vi "img_open_file.vi"(8 "error in":errorcluster, 10 "Operation (open)":enum16{"Open", "Create/Replace"}(ring), 11 "Filename":path) -> (0 "error out":errorcluster, 1 "lpBytesPerSector":u32, 2 "lpFileSize":u64, 3 "hFile":i64)   [LabVIEW 2016]
doc: "This Vi opens a file handle for unbuffered reading or writing.\n\nhFile: File handle\n\nlpFileSize: Returns the file size in bytes. Use for reading back data.\n\nlpBytesPerSector: Returns the number of bytes per sector for the hard drive array. Unbuffered reads and writes must be a multiple of the disk sector size."
uses:
  kernel32.dll
panel:
  in  "Access (read/write)":enum16{"read/write", "read-only", "write-only"}(ring)
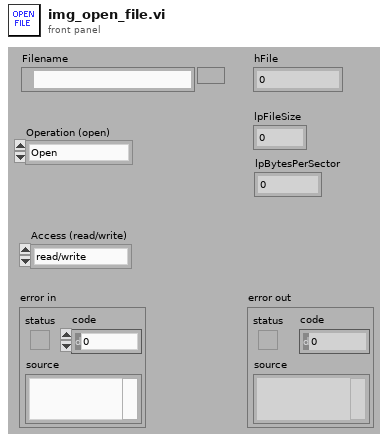
[diagram p1: front panel]
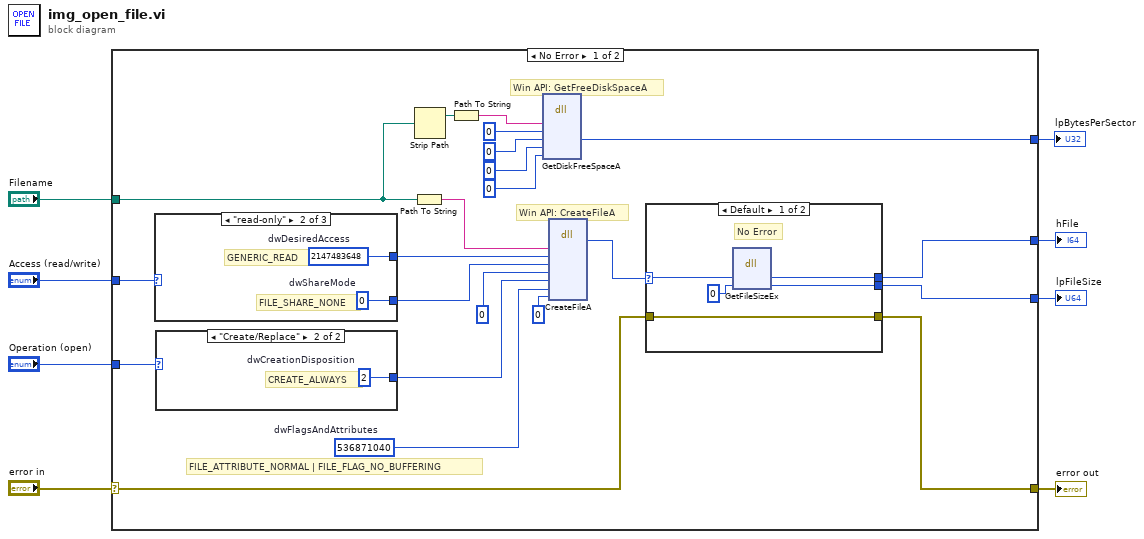
[diagram p0: block diagram]
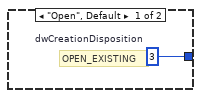
[diagram p2: hidden frame]
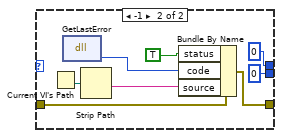
[diagram p3: hidden frame]
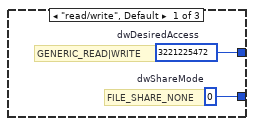
[diagram p4: hidden frame]
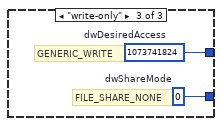
[diagram p5: hidden frame]
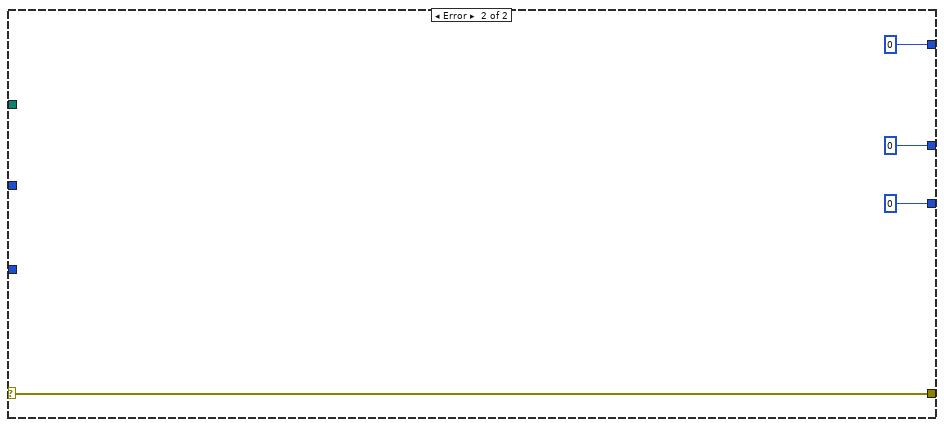
[diagram p6: hidden frame]
diagram:
  n1 = case shown="No Error" "error in" {
    selector: "error in" -> [w25 w53]
    tunnel: [w15 u32 0 ("hFile")] -> w8
    tunnel: "Filename" -> [w18 _]
    tunnel: [w26 w53] -> w6
    tunnel: "Operation (open)" -> [w11 _]
    tunnel: [w14 u64 0 ("lpFileSize")] -> w4
    tunnel: [w19 u32 0 ("lpBytesPerSector")] -> w2
    tunnel: "Access (read/write)" -> [w12 _]
    frame No Error {
      w30 = u32 536871040  # dwFlagsAndAttributes
      # "Win API: GetFreeDiskSpaceA"
      # "FILE_ATTRIBUTE_NORMAL | FILE_FLAG_NO_BUFFERING"
      # "Win API: CreateFileA"
      n2 = case shown="\"read-only\"" w12 {
        tunnel: [w46 w48 w51] -> w28
        tunnel: [w47 w49 w50] -> w27
        frame "read/write", Default {
          w46 = u32 0  # dwShareMode
          w47 = u32 3221225472  # dwDesiredAccess
          # "FILE_SHARE_NONE"
          # "GENERIC_READ|WRITE"
        }
        frame "read-only" {
          w48 = u32 0  # dwShareMode
          w49 = u32 2147483648  # dwDesiredAccess
          # "FILE_SHARE_NONE"
          # "GENERIC_READ"
        }
        frame "write-only" {
          w51 = u32 0  # dwShareMode
          w50 = u32 1073741824  # dwDesiredAccess
          # "FILE_SHARE_NONE"
          # "GENERIC_WRITE"
        }
      }
      n3 = case shown="\"Create/Replace\"" w11 {
        tunnel: [w31 w32] -> w10
        frame "Open", Default {
          w31 = u32 3  # dwCreationDisposition
          # "OPEN_EXISTING"
        }
        frame "Create/Replace" {
          w32 = u32 2  # dwCreationDisposition
          # "CREATE_ALWAYS"
        }
      }
      n4 = Path To String(path=w18) -> (string=w20:string)
      n5 = Strip Path(path=w18) -> (stripped path=w17:path)  [unwired: 1 out]
      n6 = Path To String(path=w17) -> (string=w16:string)
      n7 = dll-call lib="kernel32.dll" fn="GetDiskFreeSpaceA"("lpRootPathName"=w16, "lpSectorsPerCluster"=u32 0, "lpBytesPerSector"=u32 0, "lpNumberOfFreeClusters"=u32 0, "lpTotalNumberOfClusters"=u32 0) -> ("lpBytesPerSector"=w19:u32)  [unwired: 4 in, 6 out]
      n8 = dll-call lib="kernel32.dll" fn="CreateFileA"("lpFileName"=w20, "dwDesiredAccess"=w27, "dwShareMode"=w28, "lpSecurityAttributes"=u32 0, "dwCreationDisposition"=w10, "dwFlagsAndAttributes"=w30, "hTemplateFile"=u32 0 ("lpSecurityAttributes")) -> ("hFile"=w9:i64)  [unwired: 10 in, 2 out]
      n9 = case shown="Default" w9 {
        selector: w9 -> [w36 _]
        tunnel: w25 -> [w37 w45]
        tunnel: [w37 w44] -> w26
        tunnel: [w34 u32 0 ("hFile")] -> w15
        tunnel: [w33 u64 0 ("lpFileSize")] -> w14
        frame Default {
          # "No Error"
          n10 = dll-call lib="kernel32.dll" fn="GetFileSizeEx"("hFile"=w36, "lpFileSize"=u64 0) -> ("hFile"=w34:i64, "lpFileSize"=w33:u64)  [unwired: 3 in, 3 out]
        }
        frame -1 {
          n11 = Current VI's Path() -> (path=w42:path)
          n12 = dll-call lib="kernel32.dll" fn="GetLastError"() -> ("error"=w40:i32)  [unwired: 3 in, 2 out]
          n13 = Strip Path(path=w42) -> (name=w41:string)  [unwired: 1 out]
          n14 = Bundle By Name(cluster=w45, "status"=TRUE, "code"=w40, "source"=w41) -> (w44:errorcluster)
        }
      }
    }
    frame Error {
    }
  }
  "hFile" <- w8
  "error out" <- w6
  "lpFileSize" <- w4
  "lpBytesPerSector" <- w2
